vi "XIPIN_Gamma_Correction_7_0.vi"   [LabVIEW 2017]
doc: "The Xilinx Gamma Correction LogiCORE provides customers with a fully tested and optimized hardware block for manipulating the values of a pixel. The input video data to be adjusted for specific output display devices by applying gamma curves to be applied to each color channel independently or as a single curve to all channels. This core supports a LUT table structure, or an interpolated LUT table structure that is programmed to transform the image data for the best image quality on the display.\n------------------------------------\n<b>Need License</b> : Yes\n<b>Interface</b> : AXI4 AXI4-Stream"
uses:
  <vilib>/rvi/XilinxIP/XIPIN_XNode/niFpgaXIPIN.xnode
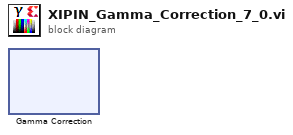
[diagram p0: block diagram]
diagram:
  n1 = xnode ("Gamma Correction")() -> ()
